vi "ADC Knob Test.vi"(0 "GEA2 Reference In":refnum<k24>, 9 "Test Results in":T1, 11 "Error In":errorcluster) -> (4 "GEA2 Reference Out":refnum<k24>, 6 "Pass/Fail?":bool, 8 "Report Text":string, 10 "Test Results out":T1, 15 "Error Out":errorcluster)   [LabVIEW 2016]
doc: "This VI performs the LED test. It first Writes the LED ERD to turn on all of the LEDs. Then prompts the user as to whether all LEDs are lit or not, for he Pass/Fail status."
uses:
  C:/Automation/DLLs/PC Dot Net/GeaCommunication.dll
  controls/Test Results.ctl
  Common/LabVIEW GEA2 Toolkit/LabVIEW_GEA2_Toolkit.lvlibp/type defs/Source_Destination.ctl
  Common/LabVIEW GEA2 Toolkit/LabVIEW_GEA2_Toolkit.lvlibp/type defs/ERD Read Data In.ctl
  Common/LabVIEW GEA2 Toolkit/LabVIEW_GEA2_Toolkit.lvlibp/type defs/Data Type.ctl
  Common/LabVIEW GEA2 Toolkit/LabVIEW_GEA2_Toolkit.lvlibp
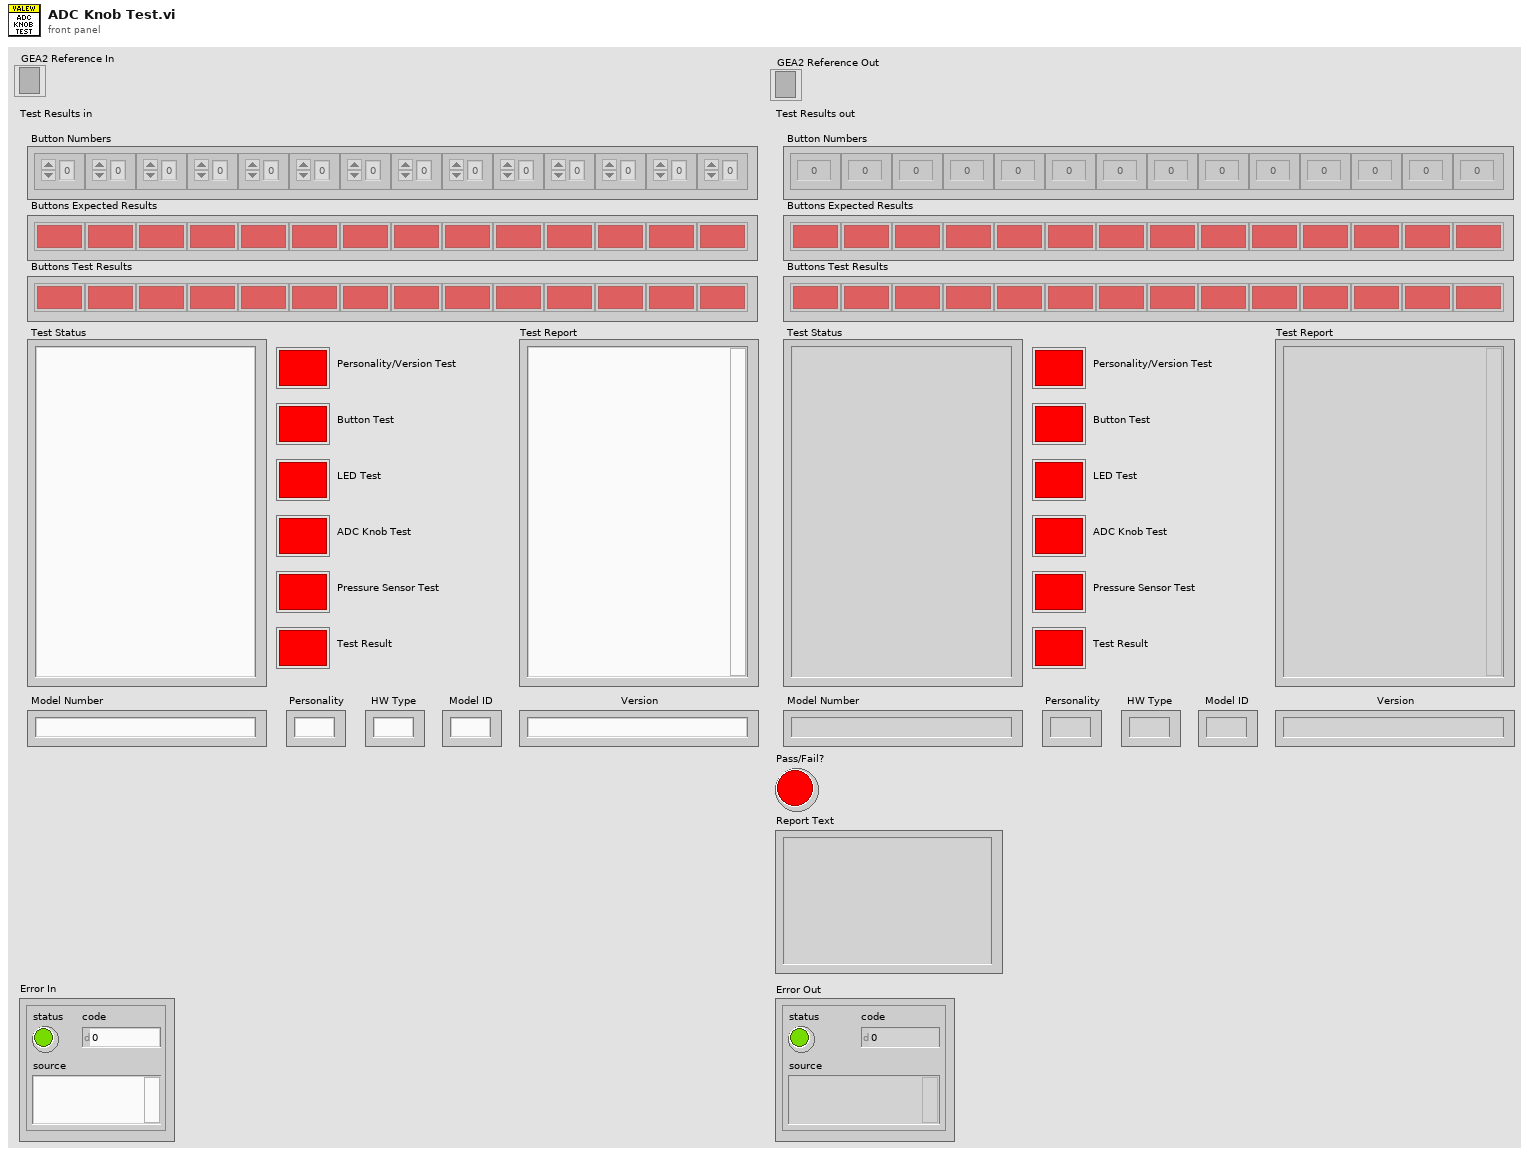
[diagram p1: front panel]
types:
  T1 = typedef "Test Results.ctl" = cluster{"Test Status":string, "Personality/Version Test ":bool, "Test Report":string, "Model Number":string, "Button Numbers":i32[], "Buttons Test Results":bool[], "Buttons Expected Results":bool[], "Model ID":string, "Personality":string, "HW Type":string, "Version":string, "Button Test":bool, "LED Test":bool, "ADC Knob Test":bool, "Pressure Sensor Test":bool, "Test Result":bool}
  T2 = typedef "LabVIEW_GEA2_Toolkit.lvlibp/ERD Read Data In.ctl" = cluster{"ERD Number":u16, "Data Type":T3}
  T3 = typedef "LabVIEW_GEA2_Toolkit.lvlibp/Data Type.ctl" = enum16{"string", "boolean", "uint8_t", "uint16_t", "uint32_t", "uint64_t", "int8_t", "int16_t", "int32_t", "int64_t"}
  T4 = typedef "LabVIEW_GEA2_Toolkit.lvlibp/Source_Destination.ctl" = cluster{"Source":u8, "Destination":u8}
  T5 = typedef "LabVIEW_GEA2_Toolkit.lvlibp/ERD Read Data Out.ctl" = cluster{"ERD Number":u16, "Data":string}
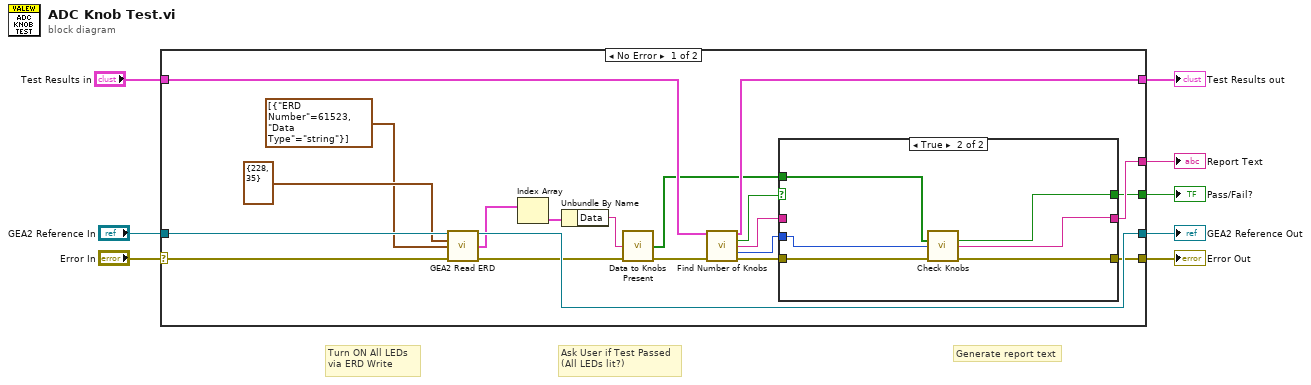
[diagram p0: block diagram]
diagram:
  # "Generate report text"
  # "Ask User if Test Passed\n(All LEDs lit?)"
  # "Turn ON All LEDs\nvia ERD Write"
  n1 = case shown="No Error" "Error In" {
    selector: "Error In" -> [w25 w40]
    tunnel: "GEA2 Reference In" -> [w28 w39]
    tunnel: [w15 w40] -> w7
    tunnel: [w26 w39] -> w6
    tunnel: "Test Results in" -> [w19 w38]
    tunnel: [w17 w38] -> w3
    tunnel: [w10 _] -> w2
    tunnel: [w9 _] -> w1
    frame No Error {
      n2 = call "GEA2 Read ERD.vi"("GEA2 Reference In"=w28, "GEA Inputs"=T4 {"Source"=228, "Destination"=35}, "Read ERD List"=T2[] [{"ERD Number"=61523, "Data Type"=enum."string"}], "Error In"=w25) -> ("GEA2 Reference Out"=w26:refnum<k24>, "ERD Data Out"=w23:T5[], "Error Out"=w21:errorcluster)  [unwired: 8 in, 1 out]
      n3 = Index Array(array=w23) -> (element=w22:T5)  [unwired: 1 in]
      n4 = Unbundle By Name(w22) -> ("Data"=w20:string)
      n5 = call "Data to Knobs Present.vi"("String"=w20, "Error In"=w21) -> ("Knobs Present"=w12:bool[], "Error Out"=w18:errorcluster)  [unwired: 12 in]
      n6 = call "Find Number of Knobs.vi"("Test Results In"=w19, "error in (no error)"=w18) -> ("Test Results Out"=w17:T1, "Pass/Fail?"=w14:bool, "Report Text"=w11:string, "Number of Knobs"=w13:i32, "error out"=w16:errorcluster)  [unwired: 9 in]
      n7 = case shown="True" w14 {
        selector: w14 -> [w29 _]
        tunnel: w16 -> [w30 w37]
        tunnel: [w30 w36] -> w15
        tunnel: w13 -> [_ w35]
        tunnel: w12 -> [_ w34]
        tunnel: w11 -> [w31 _]
        tunnel: [w31 w32] -> w10
        tunnel: [w29 w33] -> w9
        frame False {
        }
        frame True {
          n8 = call "Check Knobs.vi"("Knobs Present"=w34, "Number of Knobs"=w35, "Error In"=w37) -> ("Pass/Fail?"=w33:bool, "Report Text"=w32:string, "Error Out"=w36:errorcluster)  [unwired: 10 in]
        }
      }
    }
    frame Error {
    }
  }
  "Error Out" <- w7
  "Pass/Fail?" <- w1
  "Report Text" <- w2
  "GEA2 Reference Out" <- w6
  "Test Results out" <- w3
